vi "Main_test.vi"() -> ()   [LabVIEW 2022 SP3]
uses:
  <vilib>/DAQmx/read.llb/DAQmx Read (Analog 1D DBL NChan 1Samp).vi
  <vilib>/DAQmx/create/channels.llb/DAQmx Create Channel (AI-Voltage-Basic).vi
  <vilib>/DAQmx/miscellaneous.llb/DAQmx Fill In Error Info.vi
panel:
  in  "Boolean":bool
  out "pH value":dbl
  out "pH":dbl(knob) scale=0.0..14.0
  out "Temperature value":dbl
  out "Temperature":dbl(knob) scale=0.0..100.0
  out "Publisher Message":string
  out "Pump 1 check":bool
  out "Pump 2 check":bool
  out "Light ON/OFF":bool
  in  "stop":bool
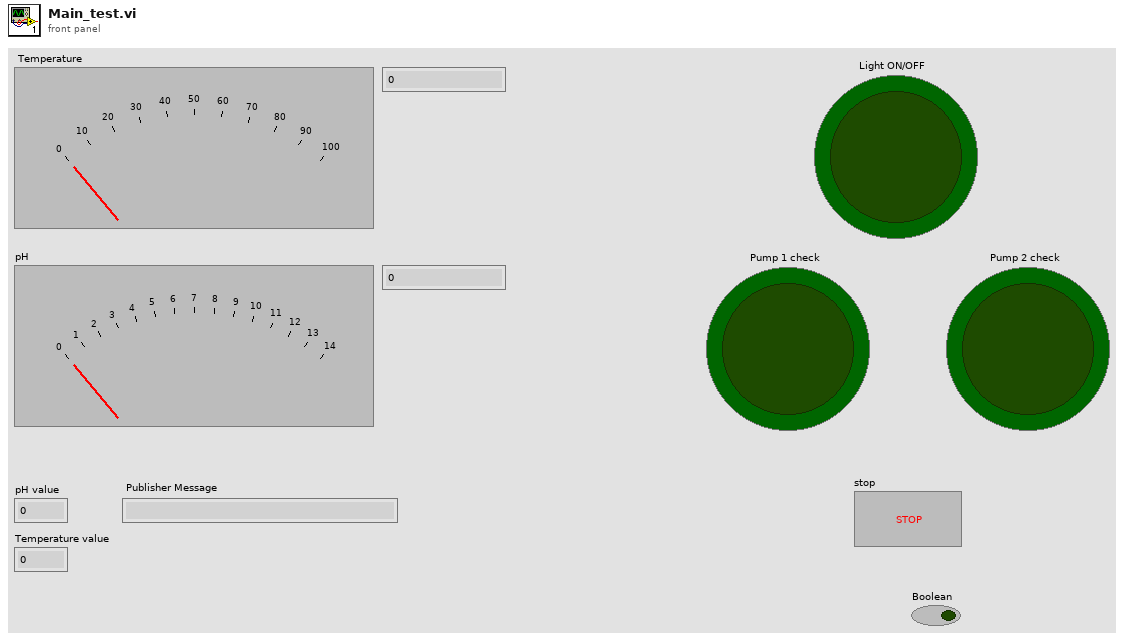
[diagram p1: front panel]
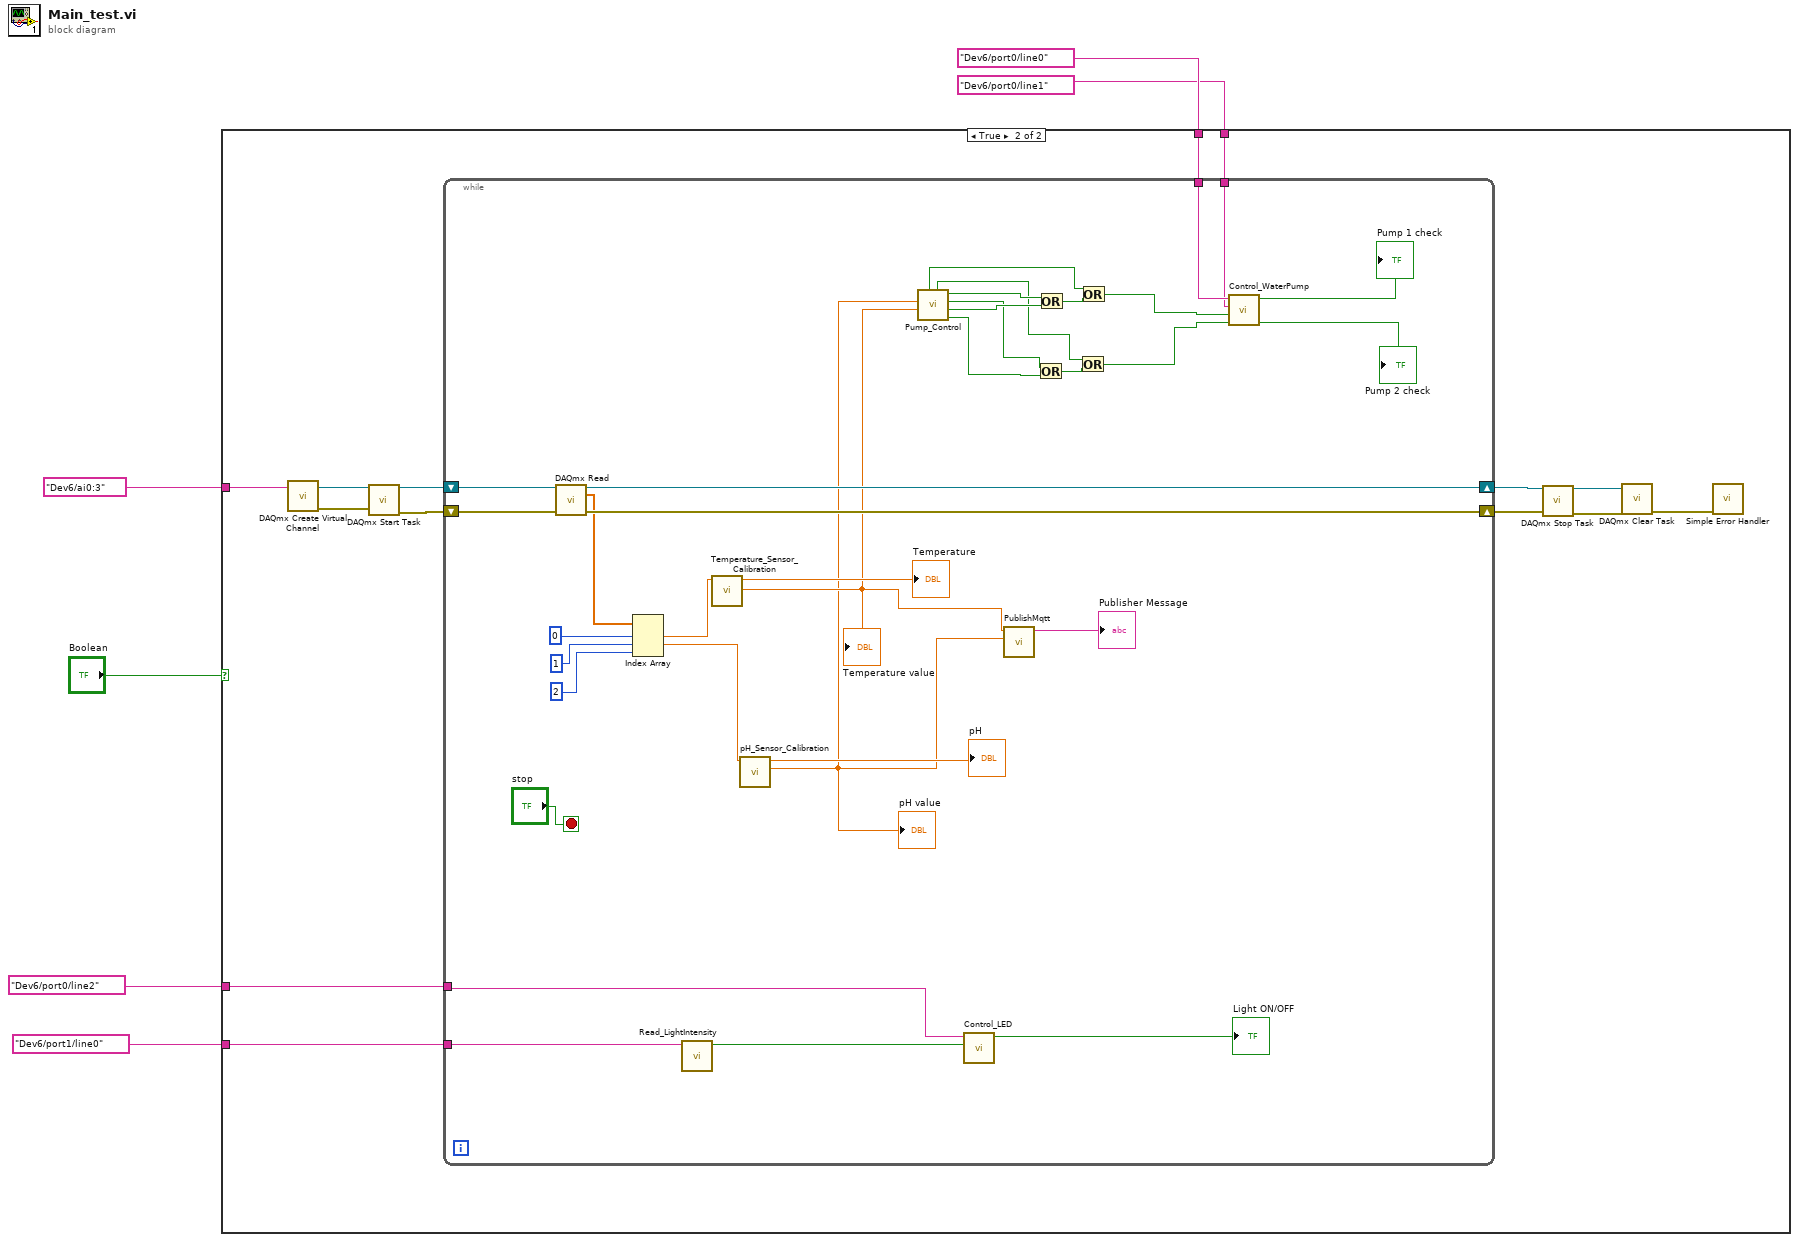
[diagram p0: block diagram]
diagram:
  n1 = case shown="True" "Boolean" {
    tunnel: tag "Dev6/ai0:3" ("physical channels") -> [_ w11]
    tunnel: tag "Dev6/port0/line0" ("Pump 1") -> [_ w10]
    tunnel: tag "Dev6/port0/line1" ("Pump 2") -> [_ w9]
    tunnel: tag "Dev6/port1/line0" ("LDR Input") -> [_ w8]
    tunnel: tag "Dev6/port0/line2" ("Light") -> [_ w7]
    frame False {
    }
    frame True {
      n2 = call-poly <vilib>:"DAQmx Create Virtual Channel.vi"("physical channels"=w11) -> ("task out"=w20:refnum<k21>, "error out"=w18:errorcluster)  [unwired: 13 in]
      n3 = call <vilib>:"DAQmx Start Task.vi"("task/channels in"=w20, "error in"=w18) -> ("task out"=w19:refnum<k21>, "error out"=w17:errorcluster)  [unwired: 12 in]
      n4 = while {
        shift-right: [w52] -> w16
        shift-left: w19 -> [w54]
        shift-right: [w51] -> w15
        shift-left: w17 -> [w53]
        tunnel: w10 -> [w27]
        tunnel: w9 -> [w26]
        tunnel: w8 -> [w24]
        tunnel: w7 -> [w22]
        stop <- "stop" stop-if-true
        n5 = call-poly <vilib>:"DAQmx Read.vi"("task/channels in"=w54, "error in"=w53) -> ("task out"=w52:refnum<k21>, "data"=w47:dbl[], "error out"=w51:errorcluster)  [unwired: 11 in]
        n6 = Index Array(array=w47, index #1=0 ("index"), index #2=1 ("index"), index #3=2 ("index")) -> (element #1=w44:dbl, element #2=w46:dbl)  [unwired: 1 out]
        n7 = call "Read_LightIntensity.vi"("LDR Input"=w24) -> ("Boolean"=w25:bool)  [unwired: 10 in]
        n8 = call "Temperature_Sensor_Calibration.vi"("read__in"=w44) -> (2:"Temperature"=w41:dbl, 3:"Temperature"=→"Temperature":dbl)  [unwired: 9 in]
        "Temperature value" <- w41
        n9 = call "pH_Sensor_Calibration.vi"("read_in"=w46) -> ("pH value"=w40:dbl, "pH"=→"pH":dbl)  [unwired: 9 in]
        "pH value" <- w40
        n10 = call "Pump_Control.vi"("Temperature"=w41, "pH"=w40) -> ("Pump 2 ON Temp"=w34:bool, "Pump 1 ON Temp"=w38:bool, "Pump 2 ON pH"=w33:bool, "Pump 1 ON pH"=w39:bool, "Pump 2 ON Water"=w32:bool, "Pump 1 ON Water"=w36:bool)  [unwired: 4 in]
        n11 = call "Control_LED.vi"("Light Signal"=w25, "Light"=w22) -> ("Light ON/OFF"=→"Light ON/OFF":bool)  [unwired: 9 in]
        n12 = call "PublishMqtt.vi"("pH"=w40, "Temp"=w41) -> ("Publisher Message"=→"Publisher Message":string)  [unwired: 9 in]
        n13 = Or(x=w33, y=w34) -> (x .or. y?=w35:bool)
        n14 = Or(x=w39, y=w38) -> (x .or. y?=w37:bool)
        n15 = Or(x=w32, y=w35) -> (x .or. y?=w30:bool)
        n16 = Or(x=w36, y=w37) -> (x .or. y?=w31:bool)
        n17 = call "Control_WaterPump.vi"("Pump 2 Signal"=w30, "Pump 1 Signal"=w31, "Pump 2"=w26, "Pump 1"=w27) -> ("Pump 2 check"=→"Pump 2 check":bool, "Pump 1 check"=→"Pump 1 check":bool)  [unwired: 6 in]
      }
      n18 = call <vilib>:"DAQmx Stop Task.vi"("task/channels in"=w16, "error in"=w15) -> ("task out"=w14:refnum<k21>, "error out"=w13:errorcluster)  [unwired: 12 in]
      n19 = call <vilib>:"DAQmx Clear Task.vi"("task in"=w14, "error in"=w13) -> ("error out"=w12:errorcluster)  [unwired: 13 in]
      n20 = call <vilib>:"Simple Error Handler.vi"("error in (no error)"=w12) -> ()  [unwired: 4 in, 5 out]
    }
  }
